vi "subDCRStatus.vi"(0 "VISA resource name":refnum<visa-resource-name>="COM2") -> (1 "VISA resource Out":refnum<visa-resource-name>="COM1", 2 "StatusCode":u8)   [LabVIEW 2012]
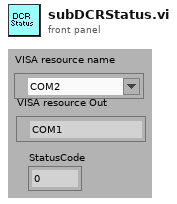
[diagram p1: front panel]
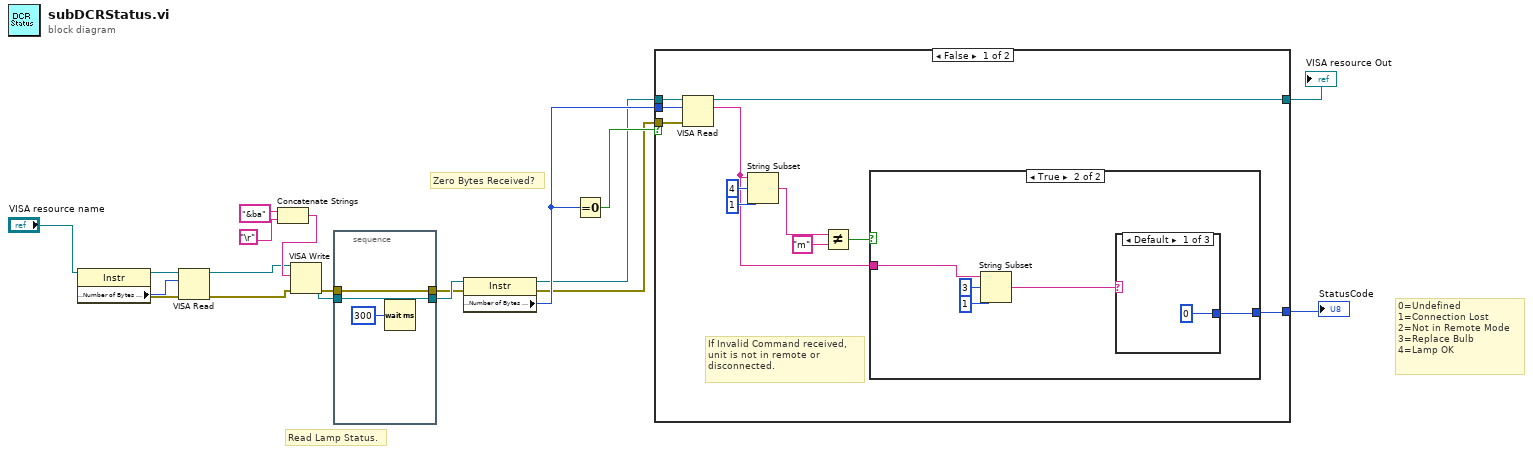
[diagram p0: block diagram]
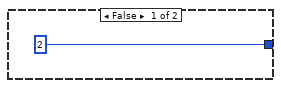
[diagram p2: hidden frame]
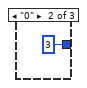
[diagram p3: hidden frame]
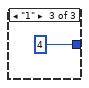
[diagram p4: hidden frame]
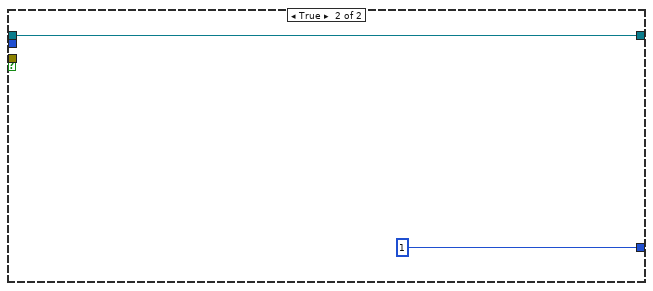
[diagram p5: hidden frame]
diagram:
  # "0=Undefined\n1=Connection Lost\n2=Not in Remote Mode\n3=Replace Bulb\n4=Lamp OK"
  # "Zero Bytes Received?"
  # "Read Lamp Status."
  n1 = property class="Instr"(reference="VISA resource name") -> (reference out=w6:refnum<visa-resource-name>, error out=w5:errorcluster, "Serial Settings:Number of Bytes at Serial Port"=w4:u32)  [unwired: 1 in]
  n2 = VISA Read(VISA resource name=w6, byte count=w4, error in (no error)=w5) -> (VISA resource name out=w2:refnum<visa-resource-name>, error out=w1:errorcluster)  [unwired: 2 out]
  n3 = Concatenate Strings("&ba" ("write buffer"), "\r") -> (w15:string)
  n4 = VISA Write(VISA resource name=w2, write buffer=w15, error in (no error)=w1) -> (VISA resource name out=w18:refnum<visa-resource-name>, error out=w13:errorcluster)  [unwired: 1 out]
  n5 = stacked-sequence {
    tunnel: w13 -> [w21]
    tunnel: [w21] -> w14
    tunnel: [w20] -> _
    tunnel: w18 -> [w20]
    frame #0 {
      n6 = Wait (ms)(milliseconds to wait=u32 300) -> ()  [unwired: 1 out]
    }
  }
  n7 = property class="Instr"(reference=w18, error in=w14) -> (reference out=w8:refnum<visa-resource-name>, error out=w10:errorcluster, "Serial Settings:Number of Bytes at Serial Port"=w11:u32)
  n8 = Equal To 0?(x=w11) -> (x = 0?=w12:bool)
  n9 = case shown="False" w12 {
    tunnel: w11 -> [w31 _]
    tunnel: w10 -> [w30 _]
    tunnel: [w29 w43] -> w9
    tunnel: w8 -> [w32 w43]
    tunnel: [w24 1] -> w7
    frame False {
      # "If Invalid Command received,\nunit is not in remote or\ndisconnected."
      n10 = VISA Read(VISA resource name=w32, byte count=w31, error in (no error)=w30) -> (VISA resource name out=w29:refnum<visa-resource-name>, read buffer=w22:string)  [unwired: 2 out]
      n11 = String Subset(string=w22, offset (0)=4, length (rest)=1 ("length (rest)")) -> (substring=w23:string)
      n12 = Not Equal?(x=w23, y="m") -> (x != y?=w25:bool)
      n13 = case shown="True" w25 {
        tunnel: [2 w38] -> w24
        tunnel: w22 -> [_ w35]
        frame False {
        }
        frame True {
          n14 = String Subset(string=w35, offset (0)=3, length (rest)=1 ("length (rest)")) -> (substring=w34:string)
          n15 = case shown="Default" w34 {
            tunnel: [0 3 4] -> w38
            frame Default {
            }
            frame "0" {
            }
            frame "1" {
            }
          }
        }
      }
    }
    frame True {
    }
  }
  "VISA resource Out" <- w9
  "StatusCode" <- w7
